vi "Start Position DAO.vi"(8 "error in (no error)":errorcluster, 9 "Displacements In":dbl[][](array[numeric]), 11 "DAO Actions":T1) -> (0 "error out":errorcluster, 1 "Displacements Out":dbl[][](array[numeric]))   [LabVIEW 2013]
uses:
  Data Access Objects/Metadata/DAO Actions.ctl
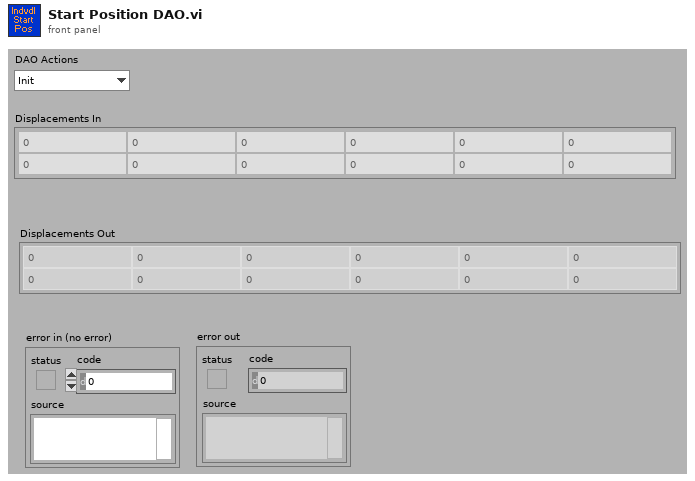
[diagram p1: front panel]
types:
  T1 = typedef "DAO Actions.ctl" = enum16{"Init", "Get", "Set"}
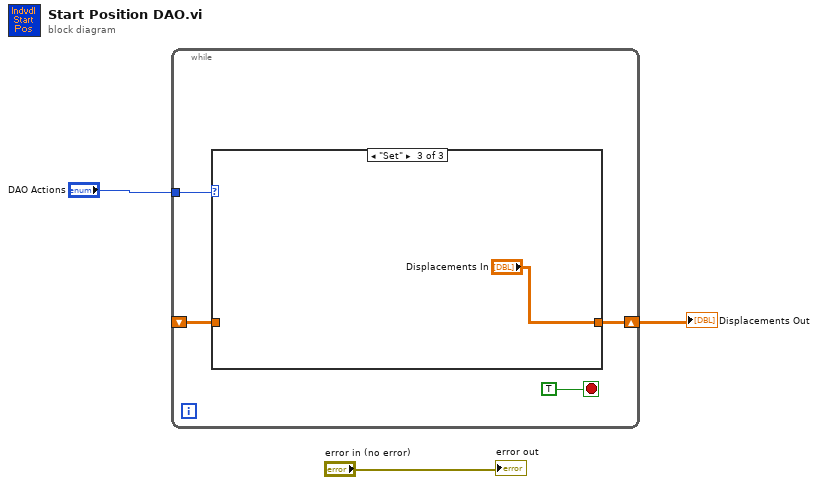
[diagram p0: block diagram]
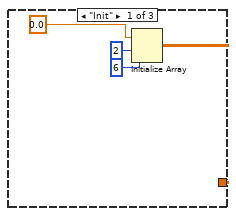
[diagram p2: hidden frame]
diagram:
  n1 = while {
    tunnel: "DAO Actions" -> [w6]
    shift-right: [w5] -> w1
    shift-left: _ -> [w4]
    stop <- TRUE stop-if-true
    n2 = case shown="\"Set\"" w6 {
      tunnel: [w8 w12 "Displacements In"] -> w5
      tunnel: w4 -> [_ w12 _]
      frame "Init" {
        n3 = Initialize Array(0.0, 2 ("dimension size"), 6 ("dimension size")) -> (w8:dbl[][])
      }
      frame "Get" {
      }
      frame "Set" {
      }
    }
  }
  "Displacements Out" <- w1
  "error out" <- "error in (no error)"
